vi "Time Converter.vi"(1 "data":string) -> (0 "time stamp":timestamp format="%<%x>T")   [LabVIEW 2015]
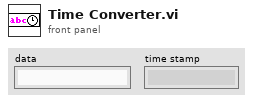
[diagram p1: front panel]
types:
  T1 = typedef "LVDateTimeRec.ctl" = cluster{"fractional second":dbl, "second":i32, "minute":i32, "hour":i32, "day of month":i32, "month":i32, "year":i32, "day of week":i32, "day of year":i32, "DST":i32}
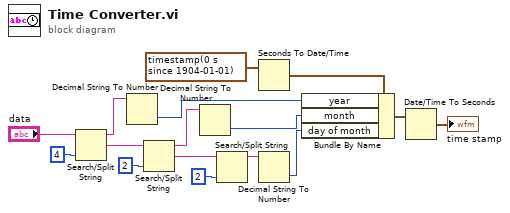
[diagram p0: block diagram]
diagram:
  n1 = Search/Split String(string="data", offset (0)=4) -> (substring before match=w8:string, match + rest of string=w13:string)  [unwired: 1 in, 1 out]
  n2 = Decimal String To Number(string=w8) -> (number=w9:i32)  [unwired: 2 in, 1 out]
  n3 = Search/Split String(string=w13, offset (0)=2) -> (substring before match=w14:string, match + rest of string=w2:string)  [unwired: 1 in, 1 out]
  n4 = Decimal String To Number(string=w14) -> (number=w15:i32)  [unwired: 2 in, 1 out]
  n5 = Search/Split String(string=w2, offset (0)=2) -> (substring before match=w1:string)  [unwired: 1 in, 2 out]
  n6 = Seconds To Date/Time(time stamp (now)=timestamp(0 s since 1904-01-01) ("time stamp")) -> (date time rec=w7:T1)  [unwired: 1 in]
  n7 = Decimal String To Number(string=w1) -> (number=w16:i32)  [unwired: 2 in, 1 out]
  n8 = Bundle By Name(cluster=w7, "year"=w9, "month"=w15, "day of month"=w16) -> (w10:T1)
  n9 = Date/Time To Seconds(2:w10) -> (0:→"time stamp":timestamp)  [unwired: 1 in]
